vi "nanocal-frontend-tcplink-client -- V2.vi"() -> ()   [LabVIEW 2020]
doc: "Demonstrates how to open a connection to an TCP server, read the data being sent, and display the data on a chart. This VI is designed to stop if the TCP connection is terminated."
uses:
  publisher action.ctl
  icicle.ctl
  array-icicle-manage-action.ctl
panel:
  out "Gamma":dbl
  out "frequency":dbl
  in  "Server Closed":string="The server VI closed the connection."
  in  "Tab Control":enum32{"Page 1", "Page 2"}(tab)
  in  "Stop":bool
  in  "address":string="146.201.231.45"
  in  "port":u16=6340
  in  "wait (ms)":u32=100
  out "nanocal data array OUT":T1[](array[typedef])
  # "nanocal tcplink --- client"
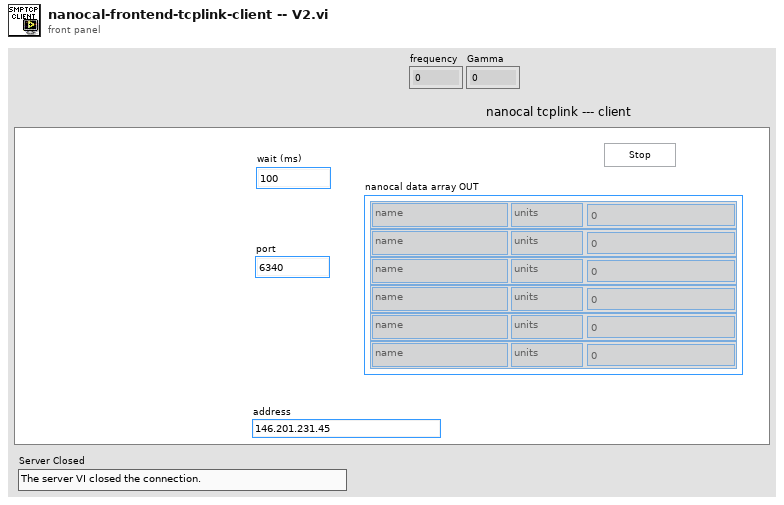
[diagram p1: front panel]
types:
  T1 = typedef "icicle.ctl" = cluster{"name":string, "units":string, "data":dbl}
  T2 = typedef "array-icicle-manage-action.ctl" = enum16{"fetch one", "fetch a few"}
  T3 = typedef "publisher action.ctl" = enum16{"set", "get", "init", "check"}
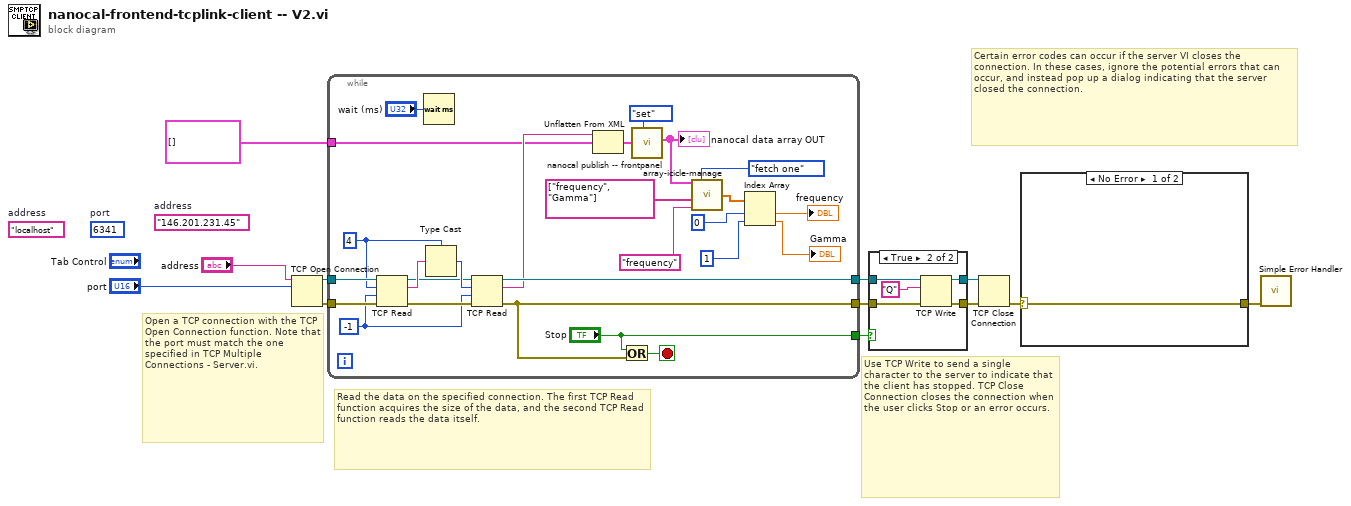
[diagram p0: block diagram]
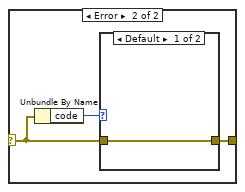
[diagram p2: hidden frame]
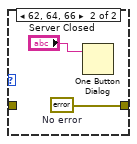
[diagram p3: hidden frame]
diagram:
  (unwired) u16 6341  # port
  (unwired) "localhost"  # address
  (unwired) "146.201.231.45"  # address
  # "Certain error codes can occur if the server VI closes the connection. In these cases, ignore the potential errors that can occur, and instead pop up a dialog indicating that the server closed the connection."
  # "Use TCP Write to send a single character to the server to indicate that the client has stopped. TCP Close Connection closes the connection when the user clicks Stop or an error occurs."
  # "Read the data on the specified connection. The first TCP Read function acquires the size of the data, and the second TCP Read function reads the data itself."
  # "Open a TCP connection with the TCP Open Connection function. Note that the port must match the one specified in TCP Multiple Connections - Server.vi."
  n1 = TCP Open Connection(address="address", remote port or service name="port") -> (connection ID=w12:refnum<k5>, error out=w11:errorcluster)  [unwired: 1 in, 2 out]
  n2 = while {
    tunnel: ["Stop"] -> w6
    tunnel: [w32] -> w10
    tunnel: [w30] -> w8
    tunnel: w11 -> [w37]
    tunnel: w12 -> [w38]
    tunnel: T1[] [] -> [w22]
    stop <- w31 stop-if-true
    w28 = -1
    w29 = 4
    n3 = TCP Read(connection ID=w38, bytes to read=w29, error in (no error)=w37, 9:w28) -> (connection ID out=w33:refnum<k5>, data out=w36:string, error out=w35:errorcluster)  [unwired: 1 out]
    n4 = Wait (ms)(milliseconds to wait="wait (ms)") -> ()  [unwired: 1 out]
    n5 = Type Cast(type=w29, x=w36) -> (*(type *) &x=w34:i32)
    n6 = TCP Read(connection ID=w33, bytes to read=w34, error in (no error)=w35, 9:w28) -> (connection ID out=w32:refnum<k5>, data out=w25:string, error out=w30:errorcluster)  [unwired: 1 out]
    n7 = Unflatten From XML(xml string=w25, type=w22) -> (value=w26:T1[])  [unwired: 1 in, 1 out]
    n8 = Or(x="Stop", y=w30) -> (x .or. y?=w31:bool)
    n9 = call "nanocal publish -- frontpanel.vi"("publisher action"=publisher_action."set", "nanocal data array IN"=w26) -> ("nanocal data array OUT"=w20:T1[])  [unwired: 9 in]
    "nanocal data array OUT" <- w20
    n10 = call "array-icicle-manage.vi"("icicle array IN"=w20, "action"=array-icicle-manage-action."fetch one", "string array IN"=string[] ["frequency", "Gamma"], "string in"="frequency") -> ("number array out"=w17:dbl[])  [unwired: 7 in, 4 out]
    n11 = Index Array(array=w17, index #1=0 ("index"), index #2=1 ("index")) -> (element #1=→"frequency":dbl, element #2=→"Gamma":dbl)
  }
  n12 = case shown="True" w6 {
    tunnel: w10 -> [w40 w45]
    tunnel: [w40 w43] -> w9
    tunnel: w8 -> [w39 w44]
    tunnel: [w39 w42] -> w7
    frame False {
    }
    frame True {
      n13 = TCP Write(connection ID=w45, data in="Q", error in (no error)=w44) -> (connection ID out=w43:refnum<k5>, error out=w42:errorcluster)  [unwired: 2 out]
    }
  }
  n14 = TCP Close Connection(connection ID=w9, error in (no error)=w7) -> (error out=w5:errorcluster)  [unwired: 2 out]
  n15 = case shown="No Error" w5 {
    selector: w5 -> [w46 w48]
    tunnel: [w46 w47] -> w4
    frame No Error {
    }
    frame Error {
      n16 = Unbundle By Name(w48) -> ("code"=w49:i32)
      n17 = case shown="Default" w49 {
        tunnel: w48 -> [w50 _]
        tunnel: [w50 w52] -> w47
        frame Default {
        }
        frame 62, 64, 66 {
          w52 = errorcluster {"status"=FALSE, "code"=0, "source"=""}  # No error
          n18 = One Button Dialog(message="Server Closed") -> ()  [unwired: 1 in, 1 out]
        }
      }
    }
  }
  n19 = call <vilib>:"Simple Error Handler.vi"("error in (no error)"=w4) -> ()  [unwired: 1 in, 8 out]
